vi "Version_4.9_8_on-chip_valves_for25ulSyringe_withModfied_Plunging.vi"() -> ()   [LabVIEW 2020] (continued)
                                frame #4 {
                                n1750 = local read "VISA Refnum in\nfor Pump"() -> (w2157:refnum<visa-resource-name>)
                                n1751 = call "PortChanger (SubVI).vi"("Port Number"="1", "VISA Refnum in"=w2157) -> ()  [unwired: 10 in]
                                }
                                frame #5 {
                                n1752 = local read "Stopper that ends \nthe main loops"() -> (w2158:bool)
                                n1753 = local read "VISA Refnum in\nfor Pump"() -> (w2159:refnum<visa-resource-name>)
                                n1754 = case shown="True" w2158 {
                                frame False {
                                }
                                frame True {
                                n1755 = local read "VISA Refnum in\nfor Pump"() -> (w2160:refnum<visa-resource-name>)
                                n1756 = call "HardStopCurrentProcess (SubVI).vi"("VISA Refnum in"=w2160) -> ()  [unwired: 11 in]
                                }
                                }
                                n1757 = call "ProcessCompletionWaiter (SubVI).vi"("VISA Refnum in"=w2159) -> ()  [unwired: 11 in]
                                }
                                frame #6 {
                                n1758 = local read "VISA Refnum in\nfor Pump"() -> (w2165:refnum<visa-resource-name>)
                                n1759 = local read "Volume of Syringe"() -> (w2162:dbl)
                                n1760 = call "GoToAbsolutePosition(SubVI).vi"("Absolute Volume Position in Syringe (in ul)"=0.0, "Volume of Syringe"=w2162, "Resolution of Pumping"=T2."Standard Pumping", "Flow Rate (ul/min)"=150.0, "VISA Refnum in"=w2165) -> ()  [unwired: 6 in, 1 out]
                                }
                                frame #7 {
                                n1761 = local read "Stopper that ends \nthe main loops"() -> (w2166:bool)
                                n1762 = local read "VISA Refnum in\nfor Pump"() -> (w2167:refnum<visa-resource-name>)
                                n1763 = case shown="True" w2166 {
                                frame False {
                                }
                                frame True {
                                n1764 = local read "VISA Refnum in\nfor Pump"() -> (w2168:refnum<visa-resource-name>)
                                n1765 = call "HardStopCurrentProcess (SubVI).vi"("VISA Refnum in"=w2168) -> ()  [unwired: 11 in]
                                }
                                }
                                n1766 = call "ProcessCompletionWaiter (SubVI).vi"("VISA Refnum in"=w2167) -> ()  [unwired: 11 in]
                                }
                                }
                                }
                              }
                            }
                          }
                          frame #19 {
                            n1767 = local read "VISA Refnum in\nfor Pump"() -> (w2170:refnum<visa-resource-name>)
                            n1768 = local read "Port for \nC2-Elution"() -> (w2169:string)
                            n1769 = call "PortChanger (SubVI).vi"("Port Number"=w2169, "VISA Refnum in"=w2170) -> ()  [unwired: 10 in]
                          }
                          frame #20 {
                            n1770 = local read "VISA Refnum in\nfor Pump"() -> (w2171:refnum<visa-resource-name>)
                            n1771 = call "ProcessCompletionWaiter (SubVI).vi"("VISA Refnum in"=w2171) -> ()  [unwired: 11 in]
                          }
                          frame #21 {
                            n1772 = local read "Buffer-C2 PickUp \nFlow Rate (ul/min)"() -> (w2175:dbl)
                            n1773 = local read "Buffer-C2 Pumping\nResolution"() -> (w2174:T2)
                            n1774 = local read "VISA Refnum in\nfor Pump"() -> (w2177:refnum<visa-resource-name>)
                            n1775 = local read "Buffer-C2 Volume \nto be Pumped"() -> (w2173:dbl)
                            n1776 = local read "Volume of Syringe"() -> (w2176:dbl)
                            n1777 = call "RPickUp(SubVI).vi"("Volume to be picked up"=w2173, "Volume of Syringe"=w2176, "Resolution of PickUP"=w2174, "PickUp Flow Rate (ul/min)"=w2175, "VISA Refnum in"=w2177) -> ()  [unwired: 6 in, 1 out]
                            n1778 = local write "SEC On"(TRUE ("SEC On")) -> ()
                          }
                          frame #22 {
                            n1779 = local read "Stopper that ends \nthe main loops"() -> (w2178:bool)
                            n1780 = local read "VISA Refnum in\nfor Pump"() -> (w2179:refnum<visa-resource-name>)
                            n1781 = case shown="True" w2178 {
                              frame False {
                              }
                              frame True {
                                n1782 = local read "VISA Refnum in\nfor Pump"() -> (w2180:refnum<visa-resource-name>)
                                n1783 = call "HardStopCurrentProcess (SubVI).vi"("VISA Refnum in"=w2180) -> ()  [unwired: 11 in]
                              }
                            }
                            n1784 = call "ProcessCompletionWaiter (SubVI).vi"("VISA Refnum in"=w2179) -> ()  [unwired: 11 in]
                          }
                          frame #23 {
                            # "Reads the initial Plunger Position for computing the volume dispensed"
                            n1785 = local read "VISA Refnum in\nfor Pump"() -> (w2182:refnum<visa-resource-name>)
                            n1786 = call "AbsolutePlungerPosition (SubVI).vi"("VISA Refnum in"=w2182) -> ("Plunger Position"=w2181:i32)  [unwired: 10 in]
                            n1787 = local write "Initial Plunger Position"(w2181) -> ()
                          }
                          frame #24 {
                            # "Switch to Port-10"
                            # "Port-10 of the pump is conncted to column-2 of chip"
                            n1788 = local read "VISA Refnum in\nfor Pump"() -> (w2184:refnum<visa-resource-name>)
                            n1789 = call "PortChanger (SubVI).vi"("Port Number"="10", "VISA Refnum in"=w2184) -> ()  [unwired: 10 in]
                          }
                          frame #25 {
                            n1790 = local read "Stopper that ends \nthe main loops"() -> (w2185:bool)
                            n1791 = local read "VISA Refnum in\nfor Pump"() -> (w2186:refnum<visa-resource-name>)
                            n1792 = case shown="True" w2185 {
                              frame False {
                              }
                              frame True {
                                n1793 = local read "VISA Refnum in\nfor Pump"() -> (w2187:refnum<visa-resource-name>)
                                n1794 = call "HardStopCurrentProcess (SubVI).vi"("VISA Refnum in"=w2187) -> ()  [unwired: 11 in]
                              }
                            }
                            n1795 = call "ProcessCompletionWaiter (SubVI).vi"("VISA Refnum in"=w2186) -> ()  [unwired: 11 in]
                          }
                          frame #26 {
                            # "Keeps the AMF valve after column-1 open and valve after column-2 closed"
                            n1796 = local read "Buffer-C2 Dispense\nFlow Rate (ul/min)"() -> (w2200:dbl)
                            n1797 = local read "Buffer-C2 Pumping\nResolution"() -> (w2199:T2)
                            n1798 = local read "VISA Refnum in\nfor Pump"() -> (w2202:refnum<visa-resource-name>)
                            n1799 = local write "Pause Data Collection"(FALSE ("Pause Data Collection")) -> ()
                            n1800 = local read "Volume of Syringe"() -> (w2201:dbl)
                            n1801 = call "GoToAbsolutePosition(SubVI).vi"("Absolute Volume Position in Syringe (in ul)"=0.0 ("Volume to be Dispensed"), "Volume of Syringe"=w2201, "Resolution of Pumping"=w2199, "Flow Rate (ul/min)"=w2200, "VISA Refnum in"=w2202) -> ()  [unwired: 6 in, 1 out]
                            n1802 = local read "VISA Refnum in\nfor Valve"() -> (w2196:refnum<visa-resource-name>)
                            n1803 = local read "External Valve \nOPEN"() -> (w2195:string)
                            n1804 = local write "Valve V1 Open"(FALSE ("Valve V1 Open")) -> ()
                            n1805 = local write "Valve V2 Open"(TRUE ("Valve V2 Open")) -> ()
                            n1806 = local write "Valve V3 Open"(TRUE ("Valve V3 Open")) -> ()
                            n1807 = local write "Valve V4 Open"(FALSE ("Valve V4 Open")) -> ()
                            n1808 = call "PortChanger_Valve (SubVI).vi"("Port Number"=w2195, "VISA Refnum in"=w2196) -> ()  [unwired: 10 in]
                            n1809 = local write "Valve V5 Open"(FALSE ("Valve V5 Open")) -> ()
                            n1810 = local write "Valve V6 Open"(FALSE ("Valve V6 Open")) -> ()
                            n1811 = local write "Valve V7 Open"(FALSE ("Valve V7 Open")) -> ()
                          }
                          frame #27 {
                            n1812 = local read "Initial Plunger Position"() -> (w2206:dbl)
                            n1813 = local read "Buffer-C2 Pumping\nResolution"() -> (w2205:T2)
                            n1814 = local read "VISA Refnum in\nfor Pump"() -> (w2207:refnum<visa-resource-name>)
                            n1815 = local read "Volume of Syringe"() -> (w2204:dbl)
                            n1816 = while {
                              tunnel: w2206 -> [w2213]
                              tunnel: w2207 -> [w2212]
                              tunnel: w2205 -> [w2211]
                              tunnel: w2204 -> [w2210]
                              stop <- w2208 stop-if-true
                              n1817 = Wait (ms)(milliseconds to wait=u32 100) -> ()  [unwired: 1 out]
                              n1818 = stacked-sequence {
                                tunnel: w2213 -> [w2219 _]
                                tunnel: w2212 -> [w2218 w2245]
                                tunnel: w2211 -> [w2217 _]
                                tunnel: w2210 -> [w2216 _]
                                tunnel: [_ w2241] -> w2208
                                frame #0 {
                                n1819 = call "AbsolutePlungerPosition (SubVI).vi"("VISA Refnum in"=w2218) -> ("Plunger Position"=w2215:i32)  [unwired: 10 in]
                                n1820 = case shown="\"Standard Pumping\", Default" w2217 {
                                tunnel: w2219 -> [w2224 w2233]
                                tunnel: w2215 -> [w2225 w2232]
                                tunnel: [w2223 w2230] -> w2214
                                tunnel: w2216 -> [w2222 w2231]
                                frame "Standard Pumping", Default {
                                n1821 = Subtract(x=w2224, y=w2225) -> (x-y=w2221:dbl)
                                n1822 = Absolute Value(x=w2221) -> (abs(x)=w2220:dbl)
                                n1823 = Multiply(x=w2220, y=w2222) -> (x*y=w2227:dbl)
                                n1824 = Divide(x=w2227, y=3000.0) -> (x/y=w2223:dbl)
                                }
                                frame "High Resolution Pumping" {
                                n1825 = Subtract(x=w2233, y=w2232) -> (x-y=w2229:dbl)
                                n1826 = Absolute Value(x=w2229) -> (abs(x)=w2228:dbl)
                                n1827 = Multiply(x=w2228, y=w2231) -> (x*y=w2235:dbl)
                                n1828 = Divide(x=w2235, y=24000.0) -> (x/y=w2230:dbl)
                                }
                                }
                                n1829 = local write "Volume being Injected \nin this process"(w2214) -> ()
                                }
                                frame #1 {
                                n1830 = local read "Stopper that ends \nthe main loops"() -> (w2242:bool)
                                n1831 = local read "Divert Buffer-C \ninto Column-2"() -> (w2243:bool)
                                n1832 = local read "Volume being Injected \nin this process"() -> (w2240:dbl)
                                n1833 = call "LSPOneStatus (SubVI).vi"("VISA Refnum in"=w2245) -> ("read buffer"=w2247:string)  [unwired: 10 in]
                                n1834 = call <vilib>:"Trim Whitespace.vi"("string"=w2247) -> ("trimmed string"=w2246:string)  [unwired: 1 in]
                                n1835 = Equal?(x=w2246, y="/0`\u0003") -> (x = y?=w2244:bool)
                                n1836 = Or(x=w2243, y=w2242) -> (x .or. y?=w2238:bool)
                                n1837 = Greater Or Equal?(x=w2240, y=2.0) -> (x >= y?=w2237:bool)
                                n1838 = Or(x=w2238, y=w2237) -> (x .or. y?=w2236:bool)
                                n1839 = Or(x=w2244, y=w2236) -> (x .or. y?=w2241:bool)
                                }
                              }
                            }
                            n1840 = local read "Stopper that ends \nthe main loops"() -> (w2203:bool)
                            n1841 = case shown="True" w2203 {
                              frame False {
                              }
                              frame True {
                                n1842 = local read "VISA Refnum in\nfor Pump"() -> (w2249:refnum<visa-resource-name>)
                                n1843 = call "HardStopCurrentProcess (SubVI).vi"("VISA Refnum in"=w2249) -> ()  [unwired: 11 in]
                              }
                            }
                          }
                          frame #28 {
                            # "Keeps the on-chip valves V4, V5 and V7 open"
                            # "Keeps the AMF valve after column-1 closed and valve after column-2 open"
                            n1844 = local write "Divert Buffer-C \ninto Column-2"(FALSE ("Divert Buffer-C \ninto Column-2")) -> ()
                            n1845 = local read "VISA Refnum in\nfor Pump"() -> (w2254:refnum<visa-resource-name>)
                            n1846 = local read "External Valve \nCLOSED"() -> (w2253:string)
                            n1847 = local write "Valve V3 Open"(FALSE ("Valve V3 Open")) -> ()
                            n1848 = local write "Valve V2 Open"(FALSE ("Valve V2 Open")) -> ()
                            n1849 = local write "Valve V1 Open"(FALSE ("Valve V1 Open")) -> ()
                            n1850 = local write "Valve V4 Open"(TRUE ("Valve V4 Open")) -> ()
                            n1851 = call "PortChanger_Valve (SubVI).vi"("Port Number"=w2253, "VISA Refnum in"=w2254) -> ()  [unwired: 10 in]
                            n1852 = local write "Valve V5 Open"(TRUE ("Valve V5 Open")) -> ()
                            n1853 = local write "Valve V6 Open"(FALSE ("Valve V6 Open")) -> ()
                            n1854 = local write "Valve V7 Open"(TRUE ("Valve V7 Open")) -> ()
                          }
                          frame #29 {
                            n1855 = local read "Initial Plunger Position"() -> (w2263:dbl)
                            n1856 = local read "Buffer-C2 Pumping\nResolution"() -> (w2262:T2)
                            n1857 = local read "VISA Refnum in\nfor Pump"() -> (w2264:refnum<visa-resource-name>)
                            n1858 = local read "Volume of Syringe"() -> (w2261:dbl)
                            n1859 = while {
                              tunnel: w2263 -> [w2270]
                              tunnel: w2264 -> [w2269]
                              tunnel: w2262 -> [w2268]
                              tunnel: w2261 -> [w2267]
                              stop <- w2265 stop-if-true
                              n1860 = Wait (ms)(milliseconds to wait=u32 100) -> ()  [unwired: 1 out]
                              n1861 = stacked-sequence {
                                tunnel: w2270 -> [w2276 _]
                                tunnel: w2269 -> [w2275 w2298]
                                tunnel: w2268 -> [w2274 _]
                                tunnel: w2267 -> [w2273 _]
                                tunnel: [_ w2296] -> w2265
                                frame #0 {
                                n1862 = call "AbsolutePlungerPosition (SubVI).vi"("VISA Refnum in"=w2275) -> ("Plunger Position"=w2272:i32)  [unwired: 10 in]
                                n1863 = case shown="\"Standard Pumping\", Default" w2274 {
                                tunnel: w2276 -> [w2281 w2290]
                                tunnel: w2272 -> [w2282 w2289]
                                tunnel: [w2280 w2287] -> w2271
                                tunnel: w2273 -> [w2279 w2288]
                                frame "Standard Pumping", Default {
                                n1864 = Subtract(x=w2281, y=w2282) -> (x-y=w2278:dbl)
                                n1865 = Absolute Value(x=w2278) -> (abs(x)=w2277:dbl)
                                n1866 = Multiply(x=w2277, y=w2279) -> (x*y=w2284:dbl)
                                n1867 = Divide(x=w2284, y=3000.0) -> (x/y=w2280:dbl)
                                }
                                frame "High Resolution Pumping" {
                                n1868 = Subtract(x=w2290, y=w2289) -> (x-y=w2286:dbl)
                                n1869 = Absolute Value(x=w2286) -> (abs(x)=w2285:dbl)
                                n1870 = Multiply(x=w2285, y=w2288) -> (x*y=w2292:dbl)
                                n1871 = Divide(x=w2292, y=24000.0) -> (x/y=w2287:dbl)
                                }
                                }
                                n1872 = local write "Volume being Injected \nin this process"(w2271) -> ()
                                }
                                frame #1 {
                                n1873 = call "LSPOneStatus (SubVI).vi"("VISA Refnum in"=w2298) -> ("read buffer"=w2300:string)  [unwired: 10 in]
                                n1874 = call <vilib>:"Trim Whitespace.vi"("string"=w2300) -> ("trimmed string"=w2299:string)  [unwired: 1 in]
                                n1875 = Equal?(x=w2299, y="/0`\u0003") -> (x = y?=w2297:bool)
                                n1876 = local read "Stopper that ends \nthe main loops"() -> (w2294:bool)
                                n1877 = local read "Divert Sample \nonto Grid"() -> (w2295:bool)
                                n1878 = Or(x=w2295, y=w2294) -> (x .or. y?=w2293:bool)
                                n1879 = Or(x=w2297, y=w2293) -> (x .or. y?=w2296:bool)
                                }
                              }
                            }
                            n1880 = local read "Stopper that ends \nthe main loops"() -> (w2260:bool)
                            n1881 = case shown="True" w2260 {
                              frame False {
                              }
                              frame True {
                                n1882 = local read "VISA Refnum in\nfor Pump"() -> (w2302:refnum<visa-resource-name>)
                                n1883 = call "HardStopCurrentProcess (SubVI).vi"("VISA Refnum in"=w2302) -> ()  [unwired: 11 in]
                              }
                            }
                          }
                          frame #30 {
                            n1884 = local read "Volume being Injected \nin this process"() -> (w2305:dbl)
                            n1885 = local read "VISA Refnum in\nfor Pump"() -> (w2307:refnum<visa-resource-name>)
                            n1886 = call "AbsolutePlungerPosition (SubVI).vi"("VISA Refnum in"=w2307) -> ("Plunger Position"=w2306:i32)  [unwired: 10 in]
                            n1887 = local write "Pause Data Collection"(TRUE) -> ()
                            n1888 = local write "True Volume being \ninjected in this\nprocess"(w2305) -> ()
                            n1889 = local write "Position\nNow"(w2306) -> ()
                            n1890 = Wait (ms)(milliseconds to wait=u32 500) -> ()  [unwired: 1 out]
                          }
                          frame #31 {
                            # "Sample Deposition onto EM-Grid"
                            n1891 = local read "Divert Sample \nonto Grid"() -> (w2308:bool)
                            n1892 = case shown="True" w2308 {
                              frame False {
                              }
                              frame True {
                                n1893 = stacked-sequence {
                                frame #0 {
                                # "Discard the initial volume of fluid that is present in the channel prior to detection"
                                n1894 = local read "Buffer-C2 Pumping\nResolution"() -> (w2319:T2)
                                n1895 = local read "Initial Plunger Position"() -> (w2318:dbl)
                                n1896 = local read "VISA Refnum in\nfor Pump"() -> (w2320:refnum<visa-resource-name>)
                                n1897 = local read "Position\nNow"() -> (w2316:dbl)
                                n1898 = local read "Volume of Syringe"() -> (w2317:dbl)
                                n1899 = local write "Pause Data Collection"(FALSE) -> ()
                                n1900 = while {
                                tunnel: w2320 -> [w2330]
                                tunnel: w2319 -> [w2329]
                                tunnel: w2318 -> [w2325]
                                tunnel: w2317 -> [w2328]
                                tunnel: w2316 -> [w2324]
                                stop <- w2326 stop-if-true
                                n1901 = stacked-sequence {
                                tunnel: w2330 -> [w2336 w2358 w2388]
                                tunnel: w2329 -> [w2335 w2357 _]
                                tunnel: w2325 -> [w2333 _ _]
                                tunnel: w2328 -> [w2332 w2355 _]
                                tunnel: [_ _ w2381] -> w2326
                                tunnel: w2324 -> [_ w2353 _]
                                frame #0 {
                                # "From here on 'True Volume being injected \nin this process' represents the true total \nvolume in this process"
                                n1902 = call "AbsolutePlungerPosition (SubVI).vi"("VISA Refnum in"=w2336) -> ("Plunger Position"=w2334:i32)  [unwired: 10 in]
                                n1903 = case shown="..\"Standard Pumping\"" w2335 {
                                tunnel: w2334 -> [w2344 w2352]
                                tunnel: w2333 -> [w2343 w2351]
                                tunnel: w2332 -> [w2340 w2348]
                                tunnel: [w2337 w2345] -> w2331
                                frame .."Standard Pumping" {
                                n1904 = Subtract(x=w2344, y=w2343) -> (x-y=w2342:dbl)
                                n1905 = Absolute Value(x=w2342) -> (abs(x)=w2341:dbl)
                                n1906 = Multiply(x=w2341, y=w2340) -> (x*y=w2339:dbl)
                                n1907 = Divide(x=w2339, y=3000.0) -> (x/y=w2337:dbl)
                                }
                                frame "High Resolution Pumping".. {
                                n1908 = Subtract(x=w2352, y=w2351) -> (x-y=w2350:dbl)
                                n1909 = Absolute Value(x=w2350) -> (abs(x)=w2349:dbl)
                                n1910 = Multiply(x=w2349, y=w2348) -> (x*y=w2347:dbl)
                                n1911 = Divide(x=w2347, y=24000.0) -> (x/y=w2345:dbl)
                                }
                                }
                                n1912 = local write "True Volume being \ninjected in this\nprocess"(w2331) -> ()
                                }
                                frame #1 {
                                # "From here on 'Volume being injected \nin this process' represents the volume \nin this sub process"
                                n1913 = call "AbsolutePlungerPosition (SubVI).vi"("VISA Refnum in"=w2358) -> ("Plunger Position"=w2356:i32)  [unwired: 10 in]
                                n1914 = case shown="..\"Standard Pumping\"" w2357 {
                                tunnel: w2356 -> [w2366 w2374]
                                tunnel: w2353 -> [w2365 w2373]
                                tunnel: w2355 -> [w2362 w2370]
                                tunnel: [w2359 w2367] -> w2354
                                frame .."Standard Pumping" {
                                n1915 = Subtract(x=w2366, y=w2365) -> (x-y=w2364:dbl)
                                n1916 = Absolute Value(x=w2364) -> (abs(x)=w2363:dbl)
                                n1917 = Multiply(x=w2363, y=w2362) -> (x*y=w2361:dbl)
                                n1918 = Divide(x=w2361, y=3000.0) -> (x/y=w2359:dbl)
                                }
                                frame "High Resolution Pumping".. {
                                n1919 = Subtract(x=w2374, y=w2373) -> (x-y=w2372:dbl)
                                n1920 = Absolute Value(x=w2372) -> (abs(x)=w2371:dbl)
                                n1921 = Multiply(x=w2371, y=w2370) -> (x*y=w2369:dbl)
                                n1922 = Divide(x=w2369, y=24000.0) -> (x/y=w2367:dbl)
                                }
                                }
                                n1923 = local write "Volume being Injected \nin this process"(w2354) -> ()
                                }
                                frame #2 {
                                n1924 = local read "Discard Volume"() -> (w2375:dbl)
                                n1925 = local read "Discard fluid \nprior to 1st \ndeposition"() -> (w2380:bool)
                                n1926 = local read "Volume being Injected \nin this process"() -> (w2379:dbl)
                                n1927 = Greater Or Equal?(x=w2379, y=w2375) -> (x >= y?=w2377:bool)
                                n1928 = call "AbsolutePlungerPositionStatus (SubVI).vi"("VISA Refnum in"=w2388) -> ("read buffer"=w2387:string)  [unwired: 10 in]
                                n1929 = local read "Stop for End of \nExperiment \nand Data Writing"() -> (w2384:bool)
                                n1930 = call <vilib>:"Trim Whitespace.vi"("string"=w2387) -> ("trimmed string"=w2386:string)  [unwired: 1 in]
                                n1931 = Not(x=w2380) -> (.not. x?=w2378:bool)
                                n1932 = Equal?(x=w2386, y="/0`\u0003") -> (x = y?=w2383:bool)
                                n1933 = Or(x=w2378, y=w2377) -> (x .or. y?=w2376:bool)
                                n1934 = Or(x=w2376, y=w2384) -> (x .or. y?=w2382:bool)
                                n1935 = Or(x=w2383, y=w2382) -> (x .or. y?=w2381:bool)
                                }
                                }
                                n1936 = Wait (ms)(milliseconds to wait=u32 100) -> ()  [unwired: 1 out]
                                }
                                n1937 = local write "Valve V4 Open"(TRUE ("Valve V4 Open")) -> ()
                                n1938 = local write "Valve V3 Open"(FALSE ("Valve V3 Open")) -> ()
                                n1939 = local write "Valve V2 Open"(FALSE ("Valve V2 Open")) -> ()
                                n1940 = local write "Valve V1 Open"(FALSE ("Valve V1 Open")) -> ()
                                n1941 = local write "Valve V5 Open"(TRUE ("Valve V5 Open")) -> ()
                                n1942 = local write "Valve V6 Open"(TRUE ("Valve V6 Open")) -> ()
                                n1943 = local write "Valve V7 Open"(FALSE ("Valve V7 Open")) -> ()
                                n1944 = local write "Volume being Injected \nin this process"(0.0) -> ()
                                }
                                frame #1 {
                                # "Keeps the on-chip valve V1, V2 and V3 closed,\nHalts also deposition onto the grid\nand waits for the 1st redeposit command. Once the command is issued\nit starts pumpoing and moves onto the next frame"
                                n1945 = stacked-sequence {
                                frame #0 {
                                n1946 = local write "Valve V5 Open"(FALSE ("Valve V5 Open")) -> ()
                                n1947 = local write "Valve V1 Open"(FALSE ("Valve V1 Open")) -> ()
                                n1948 = local read "VISA Refnum in\nfor Pump"() -> (w2398:refnum<visa-resource-name>)
                                n1949 = local write "Valve V2 Open"(FALSE ("Valve V2 Open")) -> ()
                                n1950 = local write "Valve V6 Open"(FALSE ("Valve V6 Open")) -> ()
                                n1951 = local write "Re-deposit Sample\nonto Grid"(FALSE ("Redeposit Sample\nonto Grid")) -> ()
                                n1952 = local write "Pause Data Collection"(TRUE ("Pause Data Collection")) -> ()
                                n1953 = call "HardStopCurrentProcess (SubVI).vi"("VISA Refnum in"=w2398) -> ()  [unwired: 11 in]
                                n1954 = local write "Valve V7 Open"(FALSE ("Valve V7 Open")) -> ()
                                n1955 = local write "Valve V3 Open"(FALSE ("Valve V3 Open")) -> ()
                                n1956 = local write "Valve V4 Open"(FALSE ("Valve V4 Open")) -> ()
                                }
                                frame #1 {
                                n1957 = while {
                                stop <- w2401 stop-if-true
                                n1958 = local read "Stop for End of \nExperiment \nand Data Writing"() -> (w2402:bool)
                                n1959 = local read "Re-deposit Sample\nonto Grid"() -> (w2403:bool)
                                n1960 = Or(x=w2403, y=w2402) -> (x .or. y?=w2401:bool)
                                }
                                n1961 = local write "Discard fluid \nprior to 1st \ndeposition"(FALSE ("Discard fluid \nprior to 1st \ndeposition")) -> ()
                                n1962 = One Button Dialog(message="Do you want to deposit sample on another grid? If yes, turn on 'Re-deposit Sample onto Grid'. Else turn on STOP ") -> ()  [unwired: 1 in, 1 out]
                                }
                                frame #2 {
                                n1963 = local write "Valve V6 Open"(TRUE ("Valve V3 Open")) -> ()
                                n1964 = local write "Valve V4 Open"(TRUE ("Valve V1 Open")) -> ()
                                n1965 = local write "Valve V5 Open"(TRUE ("Valve V2 Open")) -> ()
                                n1966 = local write "Valve V7 Open"(FALSE ("Valve V7 Open")) -> ()
                                }
                                frame #3 {
                                n1967 = local read "Re-deposit Sample\nonto Grid"() -> (w2408:bool)
                                n1968 = case shown="True" w2408 {
                                frame False {
                                n1969 = local write "Suction On/Off"(FALSE ("Suction On/Off")) -> ()
                                }
                                frame True {
                                n1970 = stacked-sequence {
                                frame #0 {
                                n1971 = local read "VISA Refnum in\nfor Pump"() -> (w2411:refnum<visa-resource-name>)
                                n1972 = call "AbsolutePlungerPosition (SubVI).vi"("VISA Refnum in"=w2411) -> ("Plunger Position"=w2410:i32)  [unwired: 10 in]
                                n1973 = local write "Position\nNow"(w2410) -> ()
                                }
                                frame #1 {
                                n1974 = local read "Buffer-C2 Pumping\nResolution"() -> (w2413:T2)
                                n1975 = case shown="\"Standard Pumping\", Default" w2413 {
                                tunnel: [w2414 w2425] -> w2412
                                frame "Standard Pumping", Default {
                                n1976 = local read "Buffer-C2 Volume \nto be Pumped"() -> (w2417:dbl)
                                n1977 = local read "Volume of Syringe"() -> (w2420:dbl)
                                n1978 = local read "Initial Plunger Position"() -> (w2424:dbl)
                                n1979 = local read "Position\nNow"() -> (w2423:dbl)
                                n1980 = Subtract(x=w2424, y=w2423) -> (x-y=w2422:dbl)
                                n1981 = Absolute Value(x=w2422) -> (abs(x)=w2421:dbl)
                                n1982 = Multiply(x=w2421, y=w2420) -> (x*y=w2419:dbl)
                                n1983 = Divide(x=w2419, y=3000.0) -> (x/y=w2416:dbl)
                                n1984 = Subtract(x=w2416, y=w2417) -> (x-y=w2415:dbl)
                                n1985 = Absolute Value(x=w2415) -> (abs(x)=w2414:dbl)
                                }
                                frame "High Resolution Pumping" {
                                n1986 = local read "Buffer-C2 Volume \nto be Pumped"() -> (w2428:dbl)
                                n1987 = local read "Volume of Syringe"() -> (w2431:dbl)
                                n1988 = local read "Initial Plunger Position"() -> (w2435:dbl)
                                n1989 = local read "Position\nNow"() -> (w2434:dbl)
                                n1990 = Subtract(x=w2435, y=w2434) -> (x-y=w2433:dbl)
                                n1991 = Absolute Value(x=w2433) -> (abs(x)=w2432:dbl)
                                n1992 = Multiply(x=w2432, y=w2431) -> (x*y=w2430:dbl)
                                n1993 = Divide(x=w2430, y=24000.0) -> (x/y=w2427:dbl)
                                n1994 = Subtract(x=w2427, y=w2428) -> (x-y=w2426:dbl)
                                n1995 = Absolute Value(x=w2426) -> (abs(x)=w2425:dbl)
                                }
                                }
                                n1996 = local write "Buffer-C Volume\nleft to be Pumped"(w2412) -> ()
                                }
                                frame #2 {
                                n1997 = local read "Buffer-C2 Dispense\nFlow Rate (ul/min)"() -> (w2439:dbl)
                                n1998 = local read "Buffer-C2 Pumping\nResolution"() -> (w2438:T2)
                                n1999 = local read "VISA Refnum in\nfor Pump"() -> (w2441:refnum<visa-resource-name>)
                                n2000 = local read "Volume of Syringe"() -> (w2440:dbl)
                                n2001 = call "GoToAbsolutePosition(SubVI).vi"("Absolute Volume Position in Syringe (in ul)"=0.0, "Volume of Syringe"=w2440, "Resolution of Pumping"=w2438, "Flow Rate (ul/min)"=w2439, "VISA Refnum in"=w2441) -> ()  [unwired: 6 in, 1 out]
                                n2002 = local write "Suction On/Off"(FALSE ("Suction On/Off")) -> ()
                                }
                                }
                                }
                                }
                                }
                                frame #4 {
                                n2003 = local read "Stop for End of \nExperiment \nand Data Writing"() -> (w2442:bool)
                                n2004 = case shown="True" w2442 {
                                frame False {
                                }
                                frame True {
                                n2005 = local read "VISA Refnum in\nfor Pump"() -> (w2443:refnum<visa-resource-name>)
                                n2006 = call "HardStopCurrentProcess (SubVI).vi"("VISA Refnum in"=w2443) -> ()  [unwired: 11 in]
                                }
                                }
                                }
                                }
                                }
                                frame #2 {
                                # "Keeps the on-chip valve V1, V2 Open and V3 closed"
                                n2007 = while {
                                stop <- w2447 stop-if-true
                                n2008 = local read "Suction On/Off"() -> (w2448:bool)
                                n2009 = case shown="True" w2448 {
                                frame False {
                                n2010 = local read "Buffer-C2 Pumping\nResolution"() -> (w2454:T2)
                                n2011 = local read "Initial Plunger Position"() -> (w2453:dbl)
                                n2012 = local read "VISA Refnum in\nfor Pump"() -> (w2455:refnum<visa-resource-name>)
                                n2013 = local read "Position\nNow"() -> (w2451:dbl)
                                n2014 = local read "Volume of Syringe"() -> (w2452:dbl)
                                n2015 = local write "Volume being Injected \nin this process"(0.0) -> ()
                                n2016 = local write "Pause Data Collection"(FALSE) -> ()
                                n2017 = while {
                                tunnel: w2455 -> [w2462]
                                tunnel: w2454 -> [w2461]
                                tunnel: w2453 -> [w2457]
                                tunnel: w2452 -> [w2460]
                                tunnel: w2451 -> [w2456]
                                stop <- w2458 stop-if-true
                                n2018 = stacked-sequence {
                                tunnel: w2462 -> [w2468 w2490 w2515]
                                tunnel: w2461 -> [w2467 w2489 _]
                                tunnel: w2457 -> [w2465 _ _]
                                tunnel: w2460 -> [w2464 w2487 _]
                                tunnel: [_ _ w2507] -> w2458
                                tunnel: w2456 -> [_ w2485 _]
                                frame #0 {
                                # "From here on 'True Volume being injected \nin this process' represents the true total \nvolume in this process"
                                n2019 = call "AbsolutePlungerPosition (SubVI).vi"("VISA Refnum in"=w2468) -> ("Plunger Position"=w2466:i32)  [unwired: 10 in]
                                n2020 = case shown="..\"Standard Pumping\"" w2467 {
                                tunnel: w2466 -> [w2476 w2484]
                                tunnel: w2465 -> [w2475 w2483]
                                tunnel: w2464 -> [w2472 w2480]
                                tunnel: [w2469 w2477] -> w2463
                                frame .."Standard Pumping" {
                                n2021 = Subtract(x=w2476, y=w2475) -> (x-y=w2474:dbl)
                                n2022 = Absolute Value(x=w2474) -> (abs(x)=w2473:dbl)
                                n2023 = Multiply(x=w2473, y=w2472) -> (x*y=w2471:dbl)
                                n2024 = Divide(x=w2471, y=3000.0) -> (x/y=w2469:dbl)
                                }
                                frame "High Resolution Pumping".. {
                                n2025 = Subtract(x=w2484, y=w2483) -> (x-y=w2482:dbl)
                                n2026 = Absolute Value(x=w2482) -> (abs(x)=w2481:dbl)
                                n2027 = Multiply(x=w2481, y=w2480) -> (x*y=w2479:dbl)
                                n2028 = Divide(x=w2479, y=24000.0) -> (x/y=w2477:dbl)
                                }
                                }
                                n2029 = local write "True Volume being \ninjected in this\nprocess"(w2463) -> ()
                                }
                                frame #1 {
                                # "From here on 'Volume being injected \nin this process' represents the volume \nin this sub process"
                                n2030 = call "AbsolutePlungerPosition (SubVI).vi"("VISA Refnum in"=w2490) -> ("Plunger Position"=w2488:i32)  [unwired: 10 in]
                                n2031 = case shown="..\"Standard Pumping\"" w2489 {
                                tunnel: w2488 -> [w2498 w2506]
                                tunnel: w2485 -> [w2497 w2505]
                                tunnel: w2487 -> [w2494 w2502]
                                tunnel: [w2491 w2499] -> w2486
                                frame .."Standard Pumping" {
                                n2032 = Subtract(x=w2498, y=w2497) -> (x-y=w2496:dbl)
                                n2033 = Absolute Value(x=w2496) -> (abs(x)=w2495:dbl)
                                n2034 = Multiply(x=w2495, y=w2494) -> (x*y=w2493:dbl)
                                n2035 = Divide(x=w2493, y=3000.0) -> (x/y=w2491:dbl)
                                }
                                frame "High Resolution Pumping".. {
                                n2036 = Subtract(x=w2506, y=w2505) -> (x-y=w2504:dbl)
                                n2037 = Absolute Value(x=w2504) -> (abs(x)=w2503:dbl)
                                n2038 = Multiply(x=w2503, y=w2502) -> (x*y=w2501:dbl)
                                n2039 = Divide(x=w2501, y=24000.0) -> (x/y=w2499:dbl)
                                }
                                }
                                n2040 = local write "Volume being Injected \nin this process"(w2486) -> ()
                                }
                                frame #2 {
                                n2041 = local read "Stop for End of \nExperiment \nand Data Writing"() -> (w2510:bool)
                                n2042 = local read "Suction On/Off"() -> (w2511:bool)
                                n2043 = call "AbsolutePlungerPositionStatus (SubVI).vi"("VISA Refnum in"=w2515) -> ("read buffer"=w2514:string)  [unwired: 10 in]
                                n2044 = call <vilib>:"Trim Whitespace.vi"("string"=w2514) -> ("trimmed string"=w2513:string)  [unwired: 1 in]
                                n2045 = Equal?(x=w2513, y="/0`\u0003") -> (x = y?=w2509:bool)
                                n2046 = Or(x=w2511, y=w2510) -> (x .or. y?=w2508:bool)
                                n2047 = Or(x=w2509, y=w2508) -> (x .or. y?=w2507:bool)
                                }
                                }
                                n2048 = Wait (ms)(milliseconds to wait=u32 100) -> ()  [unwired: 1 out]
                                }
                                }
                                frame True {
                                n2049 = stacked-sequence {
                                frame #0 {
                                n2050 = local read "Suction Pressure\nfor EM-grid \nDeposition (mbar)"() -> (w2520:sgl)
                                n2051 = local write "Valve V4 Open"(FALSE ("Valve V4 Open")) -> ()
                                n2052 = local read "VISA Refnum in\nfor Pump"() -> (w2523:refnum<visa-resource-name>)
                                n2053 = local write "Valve V5 Open"(FALSE ("Valve V1 Open")) -> ()
                                n2054 = local write "Suction pressure \nfor grid deposition"(w2520) -> ()
                                n2055 = local write "Re-deposit Sample\nonto Grid"(FALSE ("Redeposit Sample\nonto Grid")) -> ()
                                n2056 = local write "Pause Data Collection"(TRUE ("Pause Data Collection")) -> ()
                                n2057 = call "HardStopCurrentProcess (SubVI).vi"("VISA Refnum in"=w2523) -> ()  [unwired: 11 in]
                                n2058 = local write "Valve V6 Open"(TRUE ("Valve V2 Open")) -> ()
                                n2059 = local write "Valve V7 Open"(TRUE ("Valve V3 Open")) -> ()
                                }
                                frame #1 {
                                n2060 = call <vilib>:"fgt init.vi"() -> ("error out"=w2524:errorcluster)  [unwired: 11 in]
                                n2061 = while {
                                tunnel: [w2527] -> w2525
                                tunnel: w2524 -> [w2526]
                                stop <- w2530 stop-if-true
                                # "'5' corresponds to 2nd positin in the line-up series"
                                n2062 = local read "Stop for End of \nExperiment \nand Data Writing"() -> (w2531:bool)
                                n2063 = local read "Suction Pressure\nfor EM-grid \nDeposition (mbar)"() -> (w2528:sgl)
                                n2064 = call <vilib>:"fgt set pressure.vi"("error in (no error)"=w2526, "pressure"=w2528, "pressureIndex"=u32 1) -> ("error out"=w2527:errorcluster)  [unwired: 8 in]
                                n2065 = local read "Suction On/Off"() -> (w2533:bool)
                                n2066 = Not(x=w2533) -> (.not. x?=w2532:bool)
                                n2067 = Wait (ms)(milliseconds to wait=u32 10) -> ()  [unwired: 1 out]
                                n2068 = Or(x=w2532, y=w2531) -> (x .or. y?=w2530:bool)
                                }
                                n2069 = call <vilib>:"fgt close.vi"("error in (no error)"=w2525) -> ()  [unwired: 10 in, 1 out]
                                }
                                frame #2 {
                                n2070 = call <vilib>:"fgt init.vi"() -> ("error out"=w2536:errorcluster)  [unwired: 11 in]
                                n2071 = while {
                                tunnel: w2536 -> [w2539]
                                tunnel: [w2537] -> w2535
                                stop <- w2545 stop-if-true
                                n2072 = local read "Stop for End of \nExperiment \nand Data Writing"() -> (w2541:bool)
                                n2073 = local read "Suction On/Off"() -> (w2543:bool)
                                n2074 = call <vilib>:"fgt set pressure.vi"("error in (no error)"=w2539, "pressure"=sgl 0.0, "pressureIndex"=u32 1) -> ("error out"=w2537:errorcluster)  [unwired: 8 in]
                                n2075 = Not(x=w2543) -> (.not. x?=w2542:bool)
                                n2076 = Wait (ms)(milliseconds to wait=u32 10) -> ()  [unwired: 1 out]
                                n2077 = Or(x=w2542, y=w2541) -> (x .or. y?=w2545:bool)
                                }
                                n2078 = call <vilib>:"fgt close.vi"("error in (no error)"=w2535) -> ()  [unwired: 10 in, 1 out]
                                }
                                frame #3 {
                                n2079 = local write "Valve V7 Open"(FALSE ("Valve V3 Open")) -> ()
                                n2080 = local write "Valve V5 Open"(FALSE ("Valve V1 Open")) -> ()
                                n2081 = local write "Valve V6 Open"(FALSE ("Valve V2 Open")) -> ()
                                n2082 = local write "Valve V4 Open"(FALSE ("Valve V4 Open")) -> ()
                                }
                                frame #4 {
                                n2083 = while {
                                stop <- w2551 stop-if-true
                                n2084 = local read "Stop for End of \nExperiment \nand Data Writing"() -> (w2552:bool)
                                n2085 = local read "Re-deposit Sample\nonto Grid"() -> (w2553:bool)
                                n2086 = Or(x=w2553, y=w2552) -> (x .or. y?=w2551:bool)
                                }
                                n2087 = One Button Dialog(message="Do you want to deposit sample on another grid? If yes, turn on 'Re-deposit Sample onto Grid'. Else turn on STOP ") -> ()  [unwired: 1 in, 1 out]
                                }
                                frame #5 {
                                n2088 = local write "Valve V4 Open"(TRUE ("Valve V4 Open")) -> ()
                                n2089 = local write "Valve V7 Open"(FALSE ("Valve V3 Open")) -> ()
                                n2090 = local write "Valve V5 Open"(TRUE ("Valve V1 Open")) -> ()
                                n2091 = local write "Valve V6 Open"(TRUE ("Valve V2 Open")) -> ()
                                }
                                frame #6 {
                                n2092 = local read "Re-deposit Sample\nonto Grid"() -> (w2558:bool)
                                n2093 = case shown="False" w2558 {
                                frame False {
                                n2094 = local write "Suction On/Off"(FALSE ("Suction On/Off")) -> ()
                                }
                                frame True {
                                n2095 = stacked-sequence {
                                frame #0 {
                                n2096 = local read "VISA Refnum in\nfor Pump"() -> (w2561:refnum<visa-resource-name>)
                                n2097 = call "AbsolutePlungerPosition (SubVI).vi"("VISA Refnum in"=w2561) -> ("Plunger Position"=w2560:i32)  [unwired: 10 in]
                                n2098 = local write "Position\nNow"(w2560) -> ()
                                }
                                frame #1 {
                                n2099 = local read "Buffer-C2 Pumping\nResolution"() -> (w2563:T2)
                                n2100 = case shown="\"Standard Pumping\", Default" w2563 {
                                tunnel: [w2564 w2575] -> w2562
                                frame "Standard Pumping", Default {
                                n2101 = local read "Buffer-C2 Volume \nto be Pumped"() -> (w2567:dbl)
                                n2102 = local read "Volume of Syringe"() -> (w2570:dbl)
                                n2103 = local read "Initial Plunger Position"() -> (w2574:dbl)
                                n2104 = local read "Position\nNow"() -> (w2573:dbl)
                                n2105 = Subtract(x=w2574, y=w2573) -> (x-y=w2572:dbl)
                                n2106 = Absolute Value(x=w2572) -> (abs(x)=w2571:dbl)
                                n2107 = Multiply(x=w2571, y=w2570) -> (x*y=w2569:dbl)
                                n2108 = Divide(x=w2569, y=3000.0) -> (x/y=w2566:dbl)
                                n2109 = Subtract(x=w2566, y=w2567) -> (x-y=w2565:dbl)
                                n2110 = Absolute Value(x=w2565) -> (abs(x)=w2564:dbl)
                                }
                                frame "High Resolution Pumping" {
                                n2111 = local read "Buffer-C2 Volume \nto be Pumped"() -> (w2578:dbl)
                                n2112 = local read "Volume of Syringe"() -> (w2581:dbl)
                                n2113 = local read "Initial Plunger Position"() -> (w2585:dbl)
                                n2114 = local read "Position\nNow"() -> (w2584:dbl)
                                n2115 = Subtract(x=w2585, y=w2584) -> (x-y=w2583:dbl)
                                n2116 = Absolute Value(x=w2583) -> (abs(x)=w2582:dbl)
                                n2117 = Multiply(x=w2582, y=w2581) -> (x*y=w2580:dbl)
                                n2118 = Divide(x=w2580, y=24000.0) -> (x/y=w2577:dbl)
                                n2119 = Subtract(x=w2577, y=w2578) -> (x-y=w2576:dbl)
                                n2120 = Absolute Value(x=w2576) -> (abs(x)=w2575:dbl)
                                }
                                }
                                n2121 = local write "Buffer-C Volume\nleft to be Pumped"(w2562) -> ()
                                }
                                frame #2 {
                                n2122 = local read "Buffer-C2 Dispense\nFlow Rate (ul/min)"() -> (w2589:dbl)
                                n2123 = local read "Buffer-C2 Pumping\nResolution"() -> (w2588:T2)
                                n2124 = local read "VISA Refnum in\nfor Pump"() -> (w2591:refnum<visa-resource-name>)
                                n2125 = local read "Volume of Syringe"() -> (w2590:dbl)
                                n2126 = call "GoToAbsolutePosition(SubVI).vi"("Absolute Volume Position in Syringe (in ul)"=0.0, "Volume of Syringe"=w2590, "Resolution of Pumping"=w2588, "Flow Rate (ul/min)"=w2589, "VISA Refnum in"=w2591) -> ()  [unwired: 6 in, 1 out]
                                n2127 = local write "Suction On/Off"(FALSE ("Suction On/Off")) -> ()
                                }
                                }
                                }
                                }
                                }
                                frame #7 {
                                n2128 = local read "Stop for End of \nExperiment \nand Data Writing"() -> (w2592:bool)
                                n2129 = case shown="True" w2592 {
                                frame False {
                                }
                                frame True {
                                n2130 = local read "VISA Refnum in\nfor Pump"() -> (w2593:refnum<visa-resource-name>)
                                n2131 = call "HardStopCurrentProcess (SubVI).vi"("VISA Refnum in"=w2593) -> ()  [unwired: 11 in]
                                }
                                }
                                }
                                }
                                }
                                }
                                n2132 = local read "Stop for End of \nExperiment \nand Data Writing"() -> (w2446:bool)
                                n2133 = local read "Divert Sample \nonto Grid"() -> (w2445:bool)
                                n2134 = Not(x=w2445) -> (.not. x?=w2444:bool)
                                n2135 = Or(x=w2444, y=w2446) -> (x .or. y?=w2447:bool)
                                }
                                }
                                }
                                n2136 = local write "Discard fluid \nprior to 1st \ndeposition"(TRUE ("Discard fluid \nprior to 1st \ndeposition")) -> ()
                              }
                            }
                          }
                          frame #32 {
                            n2137 = local write "Valve V2 Open"(FALSE ("Valve V2 Open")) -> ()
                            n2138 = local write "Valve V4 Open"(FALSE ("Valve V4 Open")) -> ()
                            n2139 = local write "Valve V3 Open"(FALSE ("Valve V3 Open")) -> ()
                            n2140 = local write "Valve V1 Open"(FALSE ("Valve V1 Open")) -> ()
                            n2141 = local write "Valve V6 Open"(FALSE ("Valve V6 Open")) -> ()
                            n2142 = local write "Valve V5 Open"(FALSE ("Valve V5 Open")) -> ()
                            n2143 = local write "Valve V7 Open"(FALSE ("Valve V7 Open")) -> ()
                            n2144 = local read "VISA Refnum in\nfor Valve"() -> (w2598:refnum<visa-resource-name>)
                            n2145 = local read "External Valve \nOPEN"() -> (w2597:string)
                            n2146 = Wait (ms)(milliseconds to wait=u32 500) -> ()  [unwired: 1 out]
                            n2147 = call "PortChanger_Valve (SubVI).vi"("Port Number"=w2597, "VISA Refnum in"=w2598) -> ()  [unwired: 10 in]
                          }
                          frame #33 {
                            n2148 = local read "Stopper that ends \nthe main loops"() -> (w2605:bool)
                            n2149 = Wait (ms)(milliseconds to wait=u32 500) -> ()  [unwired: 1 out]
                            n2150 = case shown="True" w2605 {
                              frame False {
                              }
                              frame True {
                                n2151 = local read "VISA Refnum in\nfor Pump"() -> (w2609:refnum<visa-resource-name>)
                                n2152 = call "HardStopCurrentProcess (SubVI).vi"("VISA Refnum in"=w2609) -> ()  [unwired: 11 in]
                              }
                            }
                            n2153 = local write "Pause Data Collection"(TRUE ("Pause Data Collection")) -> ()
                            n2154 = local write "Start the Process"(FALSE ("Start the Process")) -> ()
                            n2155 = local write "Divert Sample \nonto Grid"(FALSE ("Divert Sample \nonto Grid")) -> ()
                          }
                          frame #34 {
                            n2156 = local write "Volume being Injected \nin this process"(0.0 ("Volume being Injected \nin this process")) -> ()
                            n2157 = local write "Elution of Column-2"(FALSE ("Elution of Column-2")) -> ()
                            n2158 = local write "SEC On"(FALSE ("SEC On")) -> ()
                          }
                        }
                      }
                    }
                  }
                }
              }
              frame True {
                n2159 = local write "Pause Data Collection"(FALSE ("Pause Data Collection")) -> ()
              }
            }
          }
          frame "Automated Plunging Alone Using Purified Protein Via Chip" {
            n2160 = local read "Stopper that ends \nthe main loops"() -> (w2614:bool)
            n2161 = case shown="False" w2614 {
              frame False {
                n2162 = local read "Start the Process"() -> (w2615:bool)
                n2163 = case shown="True" w2615 {
                  frame False {
                    n2164 = local read "Stopper that ends \nthe main loops"() -> (w2617:bool)
                    n2165 = local read "Start the Process"() -> (w2616:bool)
                    n2166 = Or(x=w2617, y=w2616) -> (x .or. y?=w2618:bool)
                    n2167 = case shown="False" w2618 {
                      frame False {
                        n2168 = while {
                          stop <- w2621 stop-if-true
                          n2169 = local read "Stop for End of \nExperiment \nand Data Writing"() -> (w2620:bool)
                          n2170 = local read "Stopper that ends \nthe main loops"() -> (w2623:bool)
                          n2171 = local read "Start the Process"() -> (w2622:bool)
                          n2172 = Wait (ms)(milliseconds to wait=u32 10) -> ()  [unwired: 1 out]
                          n2173 = Or(x=w2623, y=w2622) -> (x .or. y?=w2621:bool)
                          n2174 = local write "Stopper that ends \nthe main loops"(w2620) -> ()
                        }
                        n2175 = One Button Dialog(message="Please Select the Process and Press 'Start the Process' Button") -> ()  [unwired: 1 in, 1 out]
                      }
                      frame True {
                      }
                    }
                  }
                  frame True {
                    n2176 = stacked-sequence {
                      frame #0 {
                        # "Equilibrate Column-1 with Buffer-A obtained from port-4 and pumped via port-2 and Column-2 with Buffer-C obtained from port-4 and pumped onto chip via port-6 onto the chip ...with an initial and inbetween wash of tubings while changing the buffers"
                        n2177 = stacked-sequence {
                          frame #0 {
                            n2178 = local read "VISA Refnum in\nfor Valve"() -> (w2630:refnum<visa-resource-name>)
                            n2179 = local read "External Valve \nCLOSED"() -> (w2629:string)
                            n2180 = local write "Valve V4 Open"(FALSE ("Valve V4 Open")) -> ()
                            n2181 = local write "Valve V1 Open"(FALSE ("Valve V1 Open")) -> ()
                            n2182 = local write "Valve V2 Open"(FALSE ("Valve V2 Open")) -> ()
                            n2183 = local write "Valve V3 Open"(FALSE ("Valve V3 Open")) -> ()
                            n2184 = call "PortChanger_Valve (SubVI).vi"("Port Number"=w2629, "VISA Refnum in"=w2630) -> ()  [unwired: 10 in]
                            n2185 = local write "Valve V7 Open"(FALSE ("Valve V7 Open")) -> ()
                            n2186 = local write "Valve V5 Open"(FALSE ("Valve V5 Open")) -> ()
                            n2187 = local write "Valve V6 Open"(FALSE ("Valve V6 Open")) -> ()
                            n2188 = while {
                              stop <- w2637 stop-if-true
                              # "Keeping the valve closing pressure of push pull to zero"
                              n2189 = local read "Stop for End of \nExperiment \nand Data Writing"() -> (w2638:bool)
                              n2190 = local read "Equilibriating \nColumn-1"() -> (w2639:bool)
                              n2191 = call <vilib>:"fgt set pressure.vi"("pressure"=sgl 0.0 ("order"), "pressureIndex"=1 ("module")) -> ()  [unwired: 9 in, 1 out]
                              n2192 = Or(x=w2639, y=w2638) -> (x .or. y?=w2637:bool)
                              n2193 = Wait (ms)(milliseconds to wait=u32 10) -> ()  [unwired: 1 out]
                            }
                            n2194 = local write "Equilibriating \nColumn-1"(TRUE ("Equilibriating \nColumn-1")) -> ()
                          }
                          frame #1 {
                            # "Clean the tubing with Buffer-A1"
                            n2195 = local read "N-A1"() -> (w2641:i32)
                            n2196 = for {
                              N: w2641 -> [_]
                              n2197 = stacked-sequence {
                                frame #0 {
                                n2198 = local read "VISA Refnum in\nfor Pump"() -> (w2644:refnum<visa-resource-name>)
                                n2199 = local read "Port for \nA1-Equilibriation"() -> (w2643:string)
                                n2200 = call "PortChanger (SubVI).vi"("Port Number"=w2643, "VISA Refnum in"=w2644) -> ()  [unwired: 10 in]
                                }
                                frame #1 {
                                n2201 = local read "VISA Refnum in\nfor Pump"() -> (w2645:refnum<visa-resource-name>)
                                n2202 = call "ProcessCompletionWaiter (SubVI).vi"("VISA Refnum in"=w2645) -> ()  [unwired: 11 in]
                                }
                                frame #2 {
                                n2203 = local read "VISA Refnum in\nfor Pump"() -> (w2650:refnum<visa-resource-name>)
                                n2204 = local read "Apparent Volume\nof Syringe"() -> (w2646:dbl)
                                n2205 = local read "Volume of Syringe"() -> (w2647:dbl)
                                n2206 = call "RPickUp(SubVI).vi"("Volume to be picked up"=w2646, "Volume of Syringe"=w2647, "Resolution of PickUP"=T2."Standard Pumping", "PickUp Flow Rate (ul/min)"=150.0, "VISA Refnum in"=w2650) -> ()  [unwired: 6 in, 1 out]
                                }
                                frame #3 {
                                n2207 = local read "Stopper that ends \nthe main loops"() -> (w2651:bool)
                                n2208 = local read "VISA Refnum in\nfor Pump"() -> (w2652:refnum<visa-resource-name>)
                                n2209 = case shown="True" w2651 {
                                frame False {
                                }
                                frame True {
                                n2210 = local read "VISA Refnum in\nfor Pump"() -> (w2653:refnum<visa-resource-name>)
                                n2211 = call "HardStopCurrentProcess (SubVI).vi"("VISA Refnum in"=w2653) -> ()  [unwired: 11 in]
                                }
                                }
                                n2212 = call "ProcessCompletionWaiter (SubVI).vi"("VISA Refnum in"=w2652) -> ()  [unwired: 11 in]
                                }
                                frame #4 {
                                n2213 = local read "VISA Refnum in\nfor Pump"() -> (w2655:refnum<visa-resource-name>)
                                n2214 = call "PortChanger (SubVI).vi"("Port Number"="1", "VISA Refnum in"=w2655) -> ()  [unwired: 10 in]
                                }
                                frame #5 {
                                n2215 = local read "Stopper that ends \nthe main loops"() -> (w2656:bool)
                                n2216 = local read "VISA Refnum in\nfor Pump"() -> (w2657:refnum<visa-resource-name>)
                                n2217 = case shown="True" w2656 {
                                frame False {
                                }
                                frame True {
                                n2218 = local read "VISA Refnum in\nfor Pump"() -> (w2658:refnum<visa-resource-name>)
                                n2219 = call "HardStopCurrentProcess (SubVI).vi"("VISA Refnum in"=w2658) -> ()  [unwired: 11 in]
                                }
                                }
                                n2220 = call "ProcessCompletionWaiter (SubVI).vi"("VISA Refnum in"=w2657) -> ()  [unwired: 11 in]
                                }
                                frame #6 {
                                n2221 = local read "VISA Refnum in\nfor Pump"() -> (w2663:refnum<visa-resource-name>)
                                n2222 = local read "Volume of Syringe"() -> (w2660:dbl)
                                n2223 = call "GoToAbsolutePosition(SubVI).vi"("Absolute Volume Position in Syringe (in ul)"=0.0 ("Volume to be picked up"), "Volume of Syringe"=w2660, "Resolution of Pumping"=T2."Standard Pumping" ("Resolution of PickUP"), "Flow Rate (ul/min)"=150.0 ("PickUp Flow Rate (ul/min)"), "VISA Refnum in"=w2663) -> ()  [unwired: 6 in, 1 out]
                                }
                                frame #7 {
                                n2224 = local read "Stopper that ends \nthe main loops"() -> (w2664:bool)
                                n2225 = local read "VISA Refnum in\nfor Pump"() -> (w2665:refnum<visa-resource-name>)
                                n2226 = case shown="True" w2664 {
                                frame False {
                                }
                                frame True {
                                n2227 = local read "VISA Refnum in\nfor Pump"() -> (w2666:refnum<visa-resource-name>)
                                n2228 = call "HardStopCurrentProcess (SubVI).vi"("VISA Refnum in"=w2666) -> ()  [unwired: 11 in]
                                }
                                }
                                n2229 = call "ProcessCompletionWaiter (SubVI).vi"("VISA Refnum in"=w2665) -> ()  [unwired: 11 in]
                                }
                              }
                              n2230 = local write "Pause Data Collection"(TRUE ("Pause Data Collection")) -> ()
                            }
                          }
                          frame #2 {
                            # "Switch to Port-4"
                            # "Port-4 of pump is connected to Buffer-A1"
                            n2231 = local read "Port for \nA1-Equilibriation"() -> (w2667:string)
                            n2232 = local read "VISA Refnum in\nfor Pump"() -> (w2668:refnum<visa-resource-name>)
                            n2233 = call "PortChanger (SubVI).vi"("Port Number"=w2667, "VISA Refnum in"=w2668) -> ()  [unwired: 10 in]
                          }
                          frame #3 {
                            n2234 = local read "VISA Refnum in\nfor Pump"() -> (w2669:refnum<visa-resource-name>)
                            n2235 = call "ProcessCompletionWaiter (SubVI).vi"("VISA Refnum in"=w2669) -> ()  [unwired: 11 in]
                          }
                          frame #4 {
                            n2236 = local read "VISA Refnum in\nfor Valve"() -> (w2676:refnum<visa-resource-name>)
                            n2237 = local read "External Valve \nOPEN"() -> (w2675:string)
                            n2238 = local write "Valve V3 Open"(FALSE ("Valve V3 Open")) -> ()
                            n2239 = local write "Valve V4 Open"(FALSE ("Valve V4 Open")) -> ()
                            n2240 = local write "Valve V1 Open"(TRUE ("Valve V1 Open")) -> ()
                            n2241 = local write "Valve V2 Open"(TRUE ("Valve V2 Open")) -> ()
                            n2242 = call "PortChanger_Valve (SubVI).vi"("Port Number"=w2675, "VISA Refnum in"=w2676) -> ()  [unwired: 10 in]
                            n2243 = local write "Valve V6 Open"(FALSE ("Valve V6 Open")) -> ()
                            n2244 = local write "Valve V5 Open"(FALSE ("Valve V5 Open")) -> ()
                            n2245 = local write "Valve V7 Open"(FALSE ("Valve V7 Open")) -> ()
                          }
                          frame #5 {
                            n2246 = local read "Buffer-A1 Volume \nto be  Pumped \nfor Equilibration\nof Column-1"() -> (w2682:dbl)
                            n2247 = local read "Apparent Volume\nof Syringe"() -> (w2679:dbl)
                            n2248 = Quotient & Remainder(x=w2682, y=w2679) -> (x-y*floor(x/y)=w2680:dbl, floor(x/y)=w2681:dbl)
                            n2249 = for {
                              N: w2681 -> [_]
                              n2250 = stacked-sequence {
                                frame #0 {
                                n2251 = local read "Buffer-A1 PickUp \nFlow Rate (ul/min)\nfor Equilibration \nof Column-1"() -> (w2685:dbl)
                                n2252 = local read "Buffer-A1 Pumping\nResolution \nfor Equilibration \nof Column-1"() -> (w2684:T2)
                                n2253 = local read "VISA Refnum in\nfor Pump"() -> (w2687:refnum<visa-resource-name>)
                                n2254 = local read "Apparent Volume\nof Syringe"() -> (w2683:dbl)
                                n2255 = local read "Volume of Syringe"() -> (w2686:dbl)
